vi "ma_Check for Equality with Precision.vi"(9 "precision":i32=6, 10 "n2":dbl format="%0.17f", 11 "n1":dbl format="%0.17f") -> (0 "measured precision":i32, 1 "n1 < n2?":bool, 2 "n1 > n2?":bool, 3 "equal (within precision)":bool)   [LabVIEW 2020, in "NI_MAPro.lvlib"]
doc: "Check two floating point numbers for equality. Equality is defined as equal to precision orders of magnitude. When comparing two numbers which are supposed to be zero, if one is zero, the other must be 1E-6 or less to get equality. If both are non-zero, they are compared as usual. This may cause errors for two numbers supposed to be zero, but with round-off error so they are not zero."
uses:
  NI_MAPro.lvlib
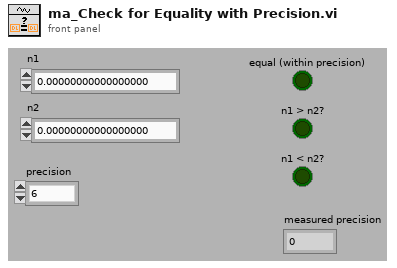
[diagram p1: front panel]
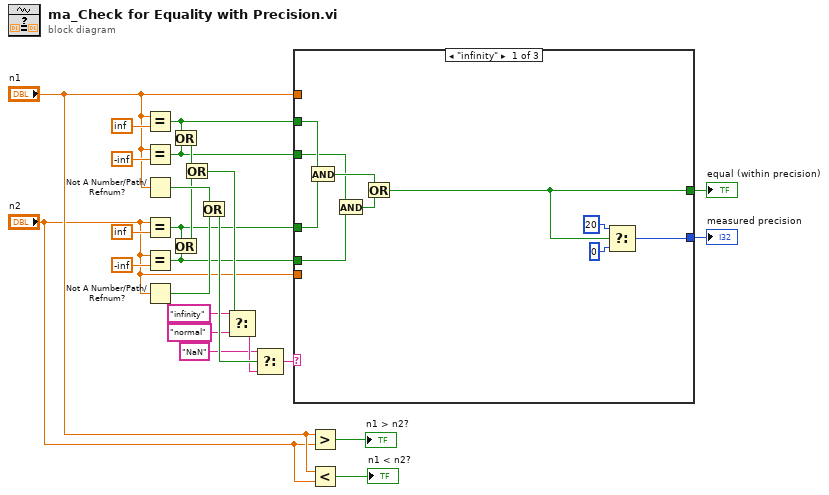
[diagram p0: block diagram]
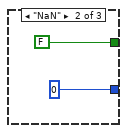
[diagram p2: hidden frame]
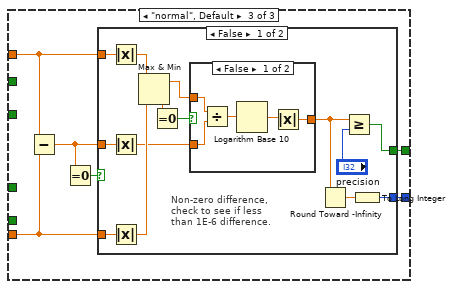
[diagram p3: hidden frame]
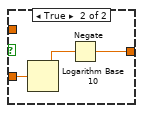
[diagram p4: hidden frame]
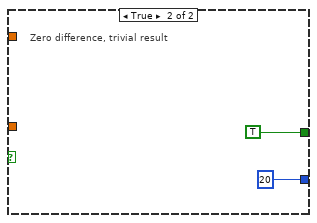
[diagram p5: hidden frame]
diagram:
  n1 = Equal?(x="n1", y=inf) -> (x = y?=w9:bool)
  n2 = Equal?(x="n1", y=-inf) -> (x = y?=w10:bool)
  n3 = Not A Number/Path/Refnum?(number/path/refnum="n1") -> (NaN/Path/Refnum?=w21:bool)
  n4 = Equal?(x="n2", y=inf) -> (x = y?=w8:bool)
  n5 = Equal?(x="n2", y=-inf) -> (x = y?=w7:bool)
  n6 = Not A Number/Path/Refnum?(number/path/refnum="n2") -> (NaN/Path/Refnum?=w20:bool)
  n7 = Or(x=w9, y=w10) -> (x .or. y?=w19:bool)
  n8 = Or(x=w8, y=w7) -> (x .or. y?=w18:bool)
  n9 = Or(x=w19, y=w18) -> (x .or. y?=w17:bool)
  n10 = Or(x=w21, y=w20) -> (x .or. y?=w16:bool)
  n11 = Select(t="infinity", s=w17, f="normal") -> (s? t:f=w15:string)
  n12 = Select(t="NaN", s=w16, f=w15) -> (s? t:f=w11:string)
  n13 = case shown="\"infinity\"" w11 {
    tunnel: [w28 FALSE w40] -> w6
    tunnel: [w29 0 w39] -> w5
    tunnel: w10 -> [w30 _ _]
    tunnel: w9 -> [w35 _ _]
    tunnel: w8 -> [w34 _ _]
    tunnel: w7 -> [w31 _ _]
    tunnel: "n1" -> [_ _ w42]
    tunnel: "n2" -> [_ _ w41]
    frame "infinity" {
      n14 = And(x=w35, y=w34) -> (x .and. y?=w33:bool)
      n15 = And(x=w30, y=w31) -> (x .and. y?=w32:bool)
      n16 = Or(x=w33, y=w32) -> (x .or. y?=w28:bool)
      n17 = Select(t=20, s=w28, f=0) -> (s? t:f=w29:i32)
    }
    frame "NaN" {
    }
    frame "normal", Default {
      n18 = Subtract(x=w42, y=w41) -> (x-y=w38:dbl)
      n19 = Equal To 0?(x=w38) -> (x = 0?=w43:bool)
      n20 = case shown="False" w43 {
        tunnel: w38 -> [w57 _]
        tunnel: w42 -> [w52 _]
        tunnel: w41 -> [w51 _]
        tunnel: [w54 TRUE] -> w40
        tunnel: [w53 20] -> w39
        frame False {
          # "Non-zero difference,\ncheck to see if less\nthan 1E-6 difference."
          n21 = Absolute Value(x=w52) -> (abs(x)=w50:dbl)
          n22 = Absolute Value(x=w57) -> (abs(x)=w44:dbl)
          n23 = Absolute Value(x=w51) -> (abs(x)=w49:dbl)
          n24 = Max & Min(x=w50, y=w49) -> (max(x,y)=w46:dbl, min(x,y)=w47:dbl)
          n25 = Equal To 0?(x=w47) -> (x = 0?=w48:bool)
          n26 = case shown="False" w48 {
            tunnel: [w62 w63] -> w55
            tunnel: w46 -> [w61 _]
            tunnel: w44 -> [w60 w65]
            frame False {
              n27 = Divide(x=w61, y=w60) -> (x/y=w59:dbl)
              n28 = Logarithm Base 10(1:w59) -> (0:w58:dbl)
              n29 = Absolute Value(x=w58) -> (abs(x)=w62:dbl)
            }
            frame True {
              n30 = Logarithm Base 10(1:w65) -> (0:w64:dbl)
              n31 = Negate(x=w64) -> (-x=w63:dbl)
            }
          }
          n32 = Round Toward -Infinity(1:w55) -> (0:w56:dbl)
          n33 = Greater Or Equal?(x=w55, y="precision") -> (x >= y?=w54:bool)
          n34 = To Long Integer(number=w56) -> (32bit integer=w53:i32)
        }
        frame True {
          # "Zero difference, trivial result"
        }
      }
    }
  }
  "measured precision" <- w5
  "equal (within precision)" <- w6
  n35 = Greater?(x="n1", y="n2") -> (0:→"n1 > n2?":bool)
  n36 = Less?(x="n1", y="n2") -> (x < y?=→"n1 < n2?":bool)
